vi "Read ALID File.vi"(8 "error in":errorcluster) -> (0 "error out":errorcluster, 3 "ALID Data":T1[](array[typedef]))   [LabVIEW 2020, in "SECS Communication.lvlib" / "SECS Data Class.lvclass"]
uses:
  SECS Data Class.lvclass
  ALID Data.ctl
  <vilib>/DATA AHEAD/XLR8/functions/Workbook/Open Create Workbook XLSX.vi
  <vilib>/DATA AHEAD/XLR8/XLR8.lvlib
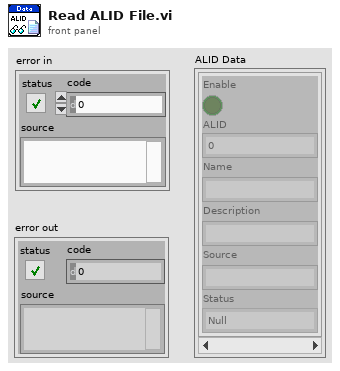
[diagram p1: front panel]
types:
  T1 = typedef "SECS Communication.lvlib/SECS Data Class.lvclass/ALID Data.ctl" = cluster{"Enable":bool, "ALID":u32, "Name":string, "Description":string, "Source":string, "Status":enum16{"Null", "Normal", "Abnormal", "Warning"}}
  T2 = typedef "XLR8.lvlib/XLR8_Ref.ctl" = cluster{"WBK":refnum<k24>, "CurSheet":refnum<k24>, "File":refnum<k24>, "file path":string, "sheet":string, "Sheets":refnum<k24>[], "IsXML":bool, "Policy":i32}
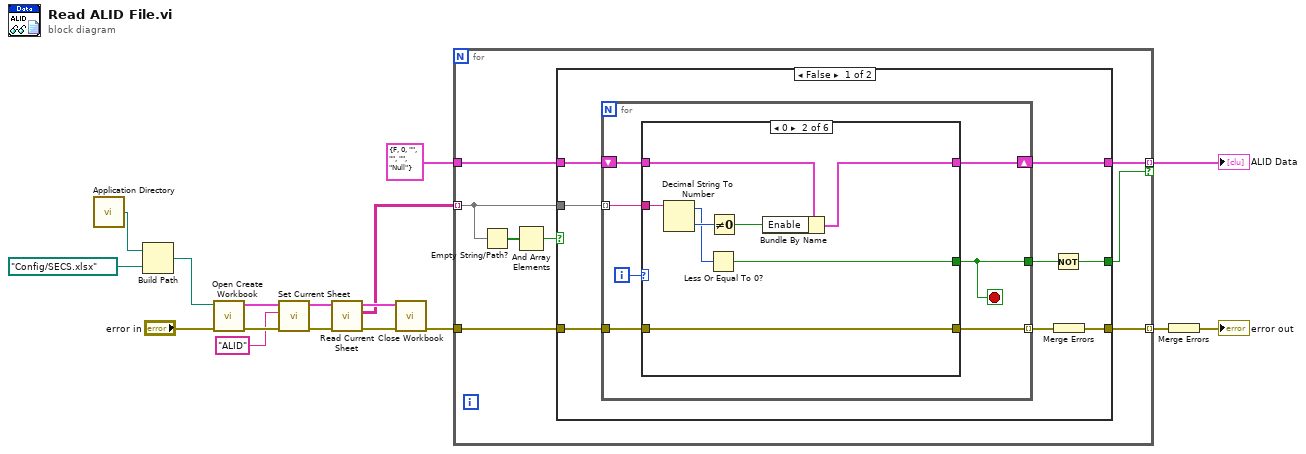
[diagram p0: block diagram]
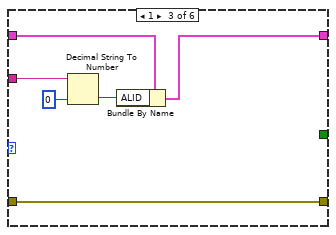
[diagram p3: hidden frame]
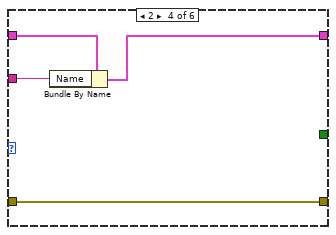
[diagram p4: hidden frame]
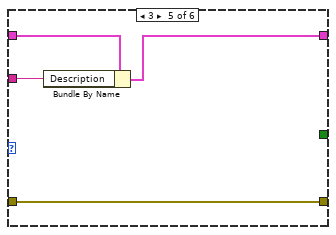
[diagram p5: hidden frame]
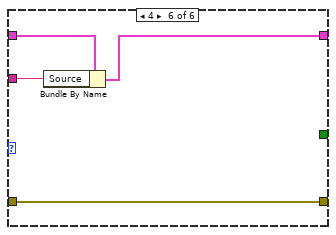
[diagram p6: hidden frame]
diagram:
  n1 = call <vilib>:"Application Directory.vi"() -> ("Application Directory"=w17:path)
  n2 = Build Path(base path=w17, name or relative path=path "Config/SECS.xlsx") -> (appended path=w14:path)
  n3 = call-poly <vilib>:"Open Create Workbook.vi"("error in"="error in", "Workbook Path"=w14) -> ("error out"=w12:errorcluster, "Refs Out"=w13:T2)  [unwired: 8 in]
  n4 = call <vilib>:"Set Current Sheet.vi"("error in"=w12, "Sheet to switch to"="ALID", "Refs In"=w13) -> ("error out"=w9:errorcluster, "Refs Out"=w10:T2)  [unwired: 7 in]
  n5 = call <vilib>:"Read Current Sheet.vi"("error in"=w9, "Refs In"=w10) -> ("error out"=w7:errorcluster, "Sheet-data out"=w5:string[][], "Refs Out"=w8:T2)  [unwired: 7 in]
  n6 = call <vilib>:"Close Workbook.vi"("error in"=w7, "Refs In"=w8) -> ("error out"=w6:errorcluster)  [unwired: 8 in, 1 out]
  n7 = for {
    tunnel: w6 -> [w22]
    tunnel: w5 -> [w23] mode=indexing
    tunnel: T1 {"Enable"=FALSE, "ALID"=0, "Name"="", "Description"="", "Source"="", "Status"=enum."Null"} ("ALID Data") -> [w21]
    tunnel: [w20] -> w1 mode=indexing if=w18
    tunnel: [w19] -> w4 mode=indexing
    n8 = Empty String/Path?(string/path=w23) -> (empty?=w25:bool[])
    n9 = And Array Elements(Boolean array=w25) -> (logical AND=w24:bool)
    n10 = case shown="False" w24 {
      tunnel: w23 -> [w33 _]
      tunnel: w22 -> [w30 w69]
      tunnel: w21 -> [w32 w70]
      tunnel: [w31 w70] -> w20
      tunnel: [w28 w69] -> w19
      tunnel: [w26 _] -> w18
      frame False {
        n11 = for {
          tunnel: w33 -> [w38] mode=indexing
          shift-right: [w37] -> w31
          shift-left: w32 -> [w40]
          tunnel: w30 -> [w36]
          tunnel: [w35] -> w29 mode=indexing
          tunnel: [w34] -> w27
          i -> [w39]
          stop <- w34 stop-if-true
          n12 = case shown="0" w39 {
            tunnel: w40 -> [w42 w47 w56 w60 w64 w67]
            tunnel: w38 -> [_ w50 w55 w59 w63 w66]
            tunnel: [w42 w45 w52 w58 w62 w68] -> w37
            tunnel: w36 -> [w41 w48 w51 w57 w61 w65]
            tunnel: [w41 w48 w51 w57 w61 w65] -> w35
            tunnel: [_ w43 _ _ _ _] -> w34
            frame Default {
            }
            frame 0 {
              n13 = Decimal String To Number(string=w50) -> (offset past number=w44:i32, number=w49:i32)  [unwired: 2 in]
              n14 = Less Or Equal To 0?(x=w44) -> (x <= 0?=w43:bool)
              n15 = Not Equal To 0?(x=w49) -> (x != 0?=w46:bool)
              n16 = Bundle By Name(cluster=w47, "Enable"=w46) -> (w45:T1)
            }
            frame 1 {
              n17 = Decimal String To Number(string=w55, default (0L)=u32 0 ("default (0 I32)")) -> (number=w54:u32)  [unwired: 1 in, 1 out]
              n18 = Bundle By Name(cluster=w56, "ALID"=w54) -> (w52:T1)
            }
            frame 2 {
              n19 = Bundle By Name(cluster=w60, "Name"=w59) -> (w58:T1)
            }
            frame 3 {
              n20 = Bundle By Name(cluster=w64, "Description"=w63) -> (w62:T1)
            }
            frame 4 {
              n21 = Bundle By Name(cluster=w67, "Source"=w66) -> (w68:T1)
            }
          }
        }
        n22 = Not(x=w27) -> (.not. x?=w26:bool)
        n23 = Merge Errors(w29) -> (w28:errorcluster)
      }
      frame True {
      }
    }
  }
  "ALID Data" <- w1
  n24 = Merge Errors(w4) -> (→"error out":errorcluster)
